vi "build.ts.vi"() -> (3 "timestampMetadata out":refnum<class "timestampMetadata.lvclass">)   [LabVIEW 2018, in "timestampMetadata.lvclass"]
uses:
  timestampMetadata.lvclass
  timestampMetadata.lvclass/timestampMetadata.ctl
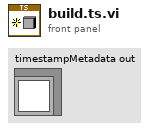
[diagram p1: front panel]
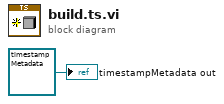
[diagram p0: block diagram]
diagram:
  "timestampMetadata out" <- refnum<class "timestampMetadata.lvclass"> refnum ("timestampMetadata in")
